vi "3D-SaveVISAParams.vi"(9 "Pic Param  Data Collect":string[][](table)=[["", "", ""], ["", "", ""]], 10 "名称或相对路径":string, 11 "路径":path) -> ()   [LabVIEW 2015]
uses:
  <vilib>/Utility/file.llb/Write To Spreadsheet File (string).vi
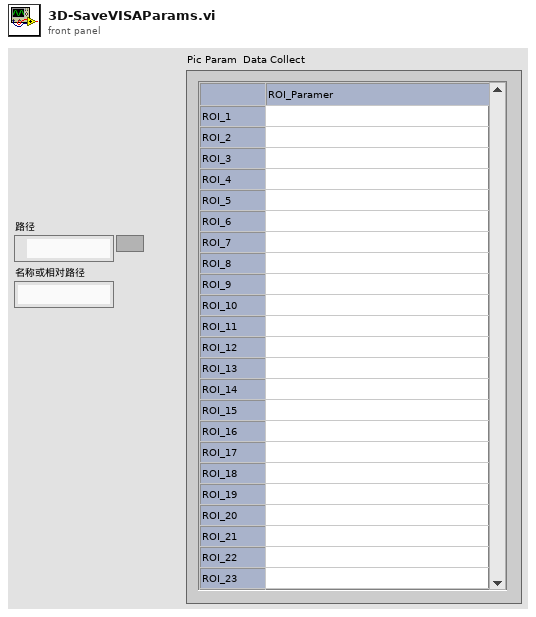
[diagram p1: front panel]
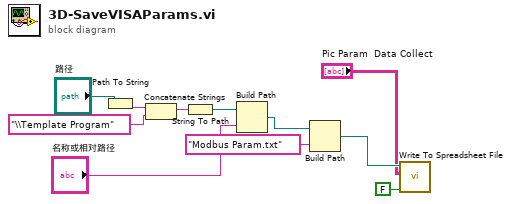
[diagram p0: block diagram]
diagram:
  n1 = Path To String(path="路径") -> (string=w11:string)
  n2 = Concatenate Strings(w11, "\\Template Program" ("字符串")) -> (w10:string)
  n3 = String To Path(string=w10) -> (path=w1:path)
  n4 = Build Path(base path=w1, name or relative path="名称或相对路径") -> (appended path=w7:path)
  n5 = Build Path(base path=w7, name or relative path="Modbus Param.txt" ("名称或相对路径")) -> (appended path=w4:path)
  n6 = call-poly <vilib>:"Write To Spreadsheet File.vi"("append to file? (new file:F)"=FALSE, "2D data"="Pic Param  Data Collect", "file path (dialog if empty)"=w4) -> ()  [unwired: 5 in, 1 out]
